vi "Open (string).vi"(6 "SQLite Library Path":path, 7 "SQLite Connection type":refnum<class "Connection.lvclass">, 8 "error in (no error)":errorcluster, 10 "busy timeout (ms)":i32=5000, 11 "db file":string) -> (0 "error out":errorcluster, 3 "SQLite Connection out":refnum<class "Connection.lvclass">)   [LabVIEW 2013, in "SQLiteSupport.lvlib" / "Connection.lvclass"]
doc: "Opens (or creates) an SQLite3 database file."
uses:
  Connection.lvclass
  Connection.lvclass/Connection.ctl
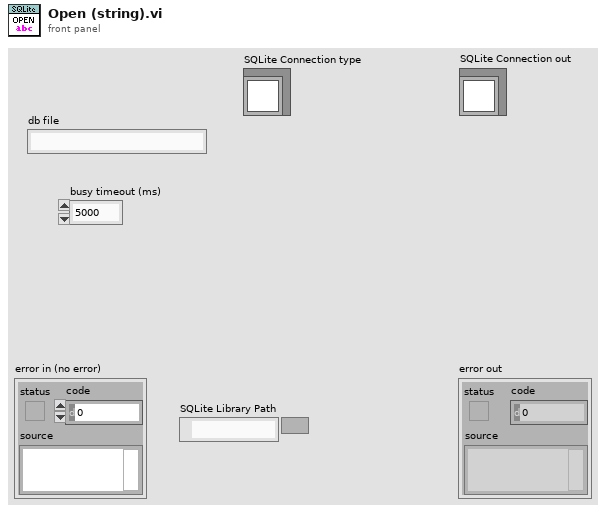
[diagram p1: front panel]
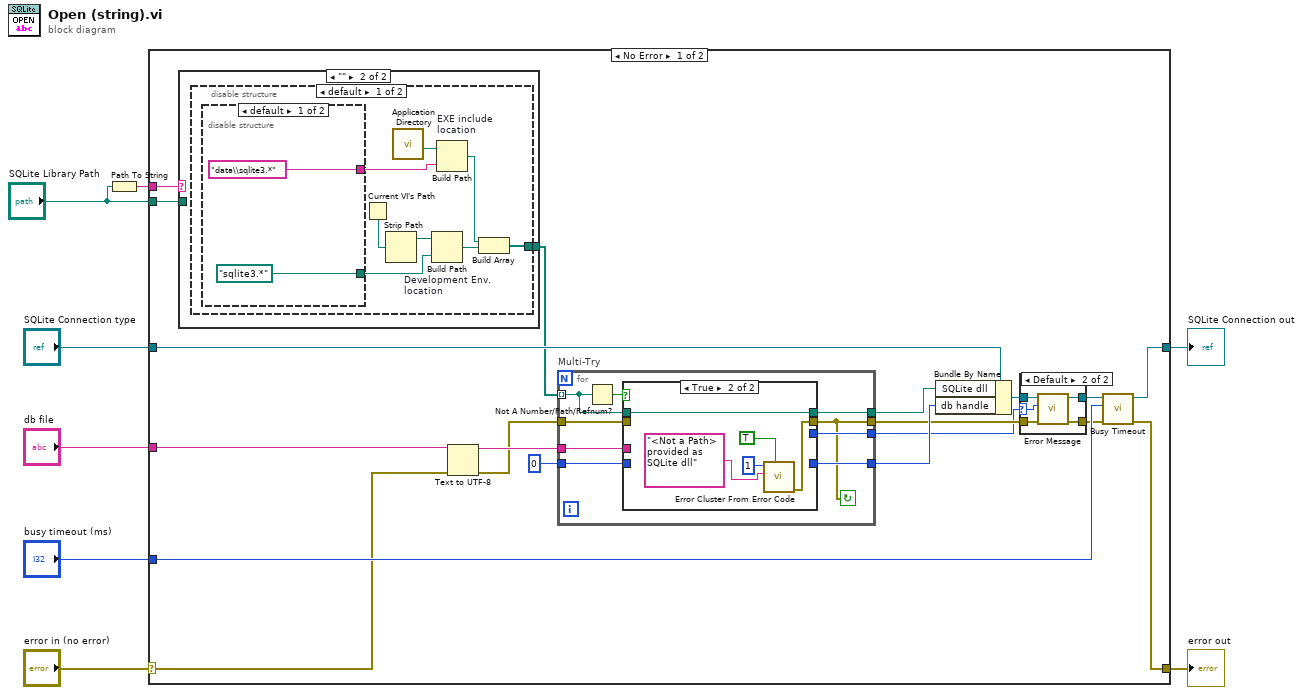
[diagram p0: block diagram]
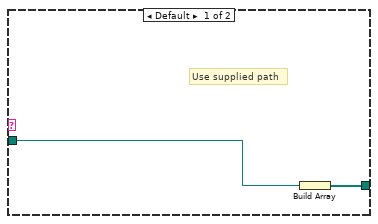
[diagram p2: hidden frame]
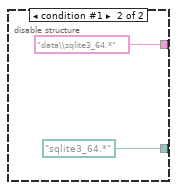
[diagram p3: hidden frame]
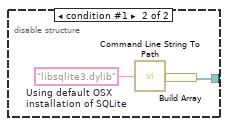
[diagram p4: hidden frame]
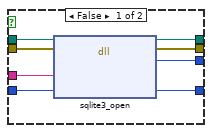
[diagram p5: hidden frame]
diagram:
  n1 = Path To String(path="SQLite Library Path") -> (string=w2:string)
  n2 = case shown="No Error" "error in (no error)" {
    selector: "error in (no error)" -> [w14 w76]
    tunnel: [w22 w76] -> w7
    tunnel: [w24 w75] -> w5
    tunnel: "SQLite Connection type" -> [w27 w75]
    tunnel: "db file" -> [w15 _]
    tunnel: "busy timeout (ms)" -> [w23 _]
    tunnel: w2 -> [w10 _]
    tunnel: "SQLite Library Path" -> [w9 _]
    frame No Error {
      n3 = case shown="\"\"" w10 {
        tunnel: [w28 w30] -> w21
        tunnel: w9 -> [w29 _]
        frame Default {
          # "Use supplied path"
          n4 = Build Array(w29) -> (w28:path[])
        }
        frame "" {
          n5 = disable-structure shown="default" {
            disable-tunnel: [w35 w43] -> w30
            frame condition #0 (active) {
              n6 = disable-structure shown="default" {
                disable-tunnel: ["data\\sqlite3.*" ("name or relative path") "data\\sqlite3_64.*" ("name or relative path")] -> w37
                disable-tunnel: [path "sqlite3.*" ("Application Directory") path "sqlite3_64.*" ("Application Directory")] -> w32
                frame condition #0 (active) {
                }
                frame condition #1 {
                }
              }
              n7 = Current VI's Path() -> (path=w34:path)
              n8 = Strip Path(path=w34) -> (stripped path=w33:path)  [unwired: 1 out]
              n9 = call <vilib>:"Application Directory.vi"() -> ("Application Directory"=w36:path)
              n10 = Build Path "Development Env.\nlocation"(base path=w33, name or relative path=w32) -> (appended path=w31:path)
              n11 = Build Path "EXE include\nlocation"(base path=w36, name or relative path=w37) -> (appended path=w38:path)
              n12 = Build Array(w38, w31) -> (w35:path[])
            }
            frame condition #1 {
              w44 = "libsqlite3.dylib"  # Using default OSX installation of SQLite
              n13 = call <vilib>:"Command Line String To Path.vi"("string"=w44) -> ("path"=w45:path)
              n14 = Build Array(w45) -> (w43:path[])
            }
          }
        }
      }
      n15 = Text to UTF-8(8:w14, 11:w15) -> (0:w11:errorcluster, 3:w12:string)
      n16 = for "Multi-Try" {
        tunnel: u64 0 ("handle") -> [w54]
        tunnel: [w53] -> w18
        tunnel: [w48] -> w20
        tunnel: [w52] -> w26
        tunnel: [w51] -> w25
        tunnel: w11 -> [w49]
        tunnel: w21 -> [w47] mode=indexing
        tunnel: w12 -> [w50]
        stop <- w48 continue-if-true
        n17 = Not A Number/Path/Refnum?(number/path/refnum=w47) -> (NaN/Path/Refnum?=w46:bool)
        n18 = case shown="True" w46 {
          tunnel: w54 -> [w62 _]
          tunnel: [w61 _] -> w53
          tunnel: [w60 _] -> w52
          tunnel: [w59 w67] -> w51
          tunnel: w50 -> [w58 _]
          tunnel: w49 -> [w57 _]
          tunnel: [w56 w66] -> w48
          tunnel: w47 -> [w55 w67]
          frame False {
            n19 = dll-call lib="C:/LabVIEW_JDP/Support/SQLite/SQL Connection/sqlite3.dll" fn="sqlite3_open"(path in=w55, error in=w57, "File"=w58, "db handle"=w62) -> (path out=w59:path, error out=w56:errorcluster, "return type"=w61:i32, "db handle"=w60:u64)  [unwired: 2 in]
          }
          frame True {
            n20 = call <vilib>:"Error Cluster From Error Code.vi"("show call chain? (False)"=TRUE, "error message (\"\")"="<Not a Path> provided as SQLite dll" ("source"), "error code (0)"=1) -> ("error out"=w66:errorcluster)  [unwired: 6 in]
          }
        }
      }
      n21 = Bundle By Name(cluster=w27, "SQLite dll"=w25, "db handle"=w26) -> (w19:refnum<class "Connection.lvclass">)
      n22 = case shown="Default" w18 {
        selector: w18 -> [_ w70]
        tunnel: w19 -> [w69 w74]
        tunnel: [w69 w73] -> w17
        tunnel: w20 -> [w68 w72]
        tunnel: [w68 w71] -> w16
        frame 0 {
          # "No Error"
        }
        frame Default {
          n23 = call "Error Message.vi"("error in (no error)"=w72, "error code"=w70, "Connection in"=w74) -> ("error out"=w71:errorcluster, "Connection out"=w73:refnum<class "Connection.lvclass">)  [unwired: 7 in]
        }
      }
      n24 = call "Busy Timeout.vi"("error in (no error)"=w16, "busy timeout (ms)"=w23, "Connection in"=w17) -> ("error out"=w22:errorcluster, "Connection out"=w24:refnum<class "Connection.lvclass">)  [unwired: 7 in]
    }
    frame Error {
    }
  }
  "error out" <- w7
  "SQLite Connection out" <- w5
